vi "vipUninstall.vi"() -> ()   [LabVIEW 2014, in "lv-cli-steps.lvlib"]
uses:
  lv-cli-steps.lvlib
  <vilib>/Utility/error.llb/DialogType.ctl
  <vilib>/Wiresmith Technology/LabVIEW CLI/CLI Class/CLI.lvclass
  <vilib>/JKI/VIPM API/VIPM API_vipm_api.lvlib
panel:
  out "error out":errorcluster
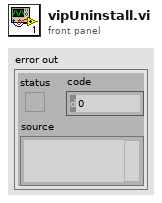
[diagram p1: front panel]
types:
  T1 = typedef "DialogType.ctl" = u16
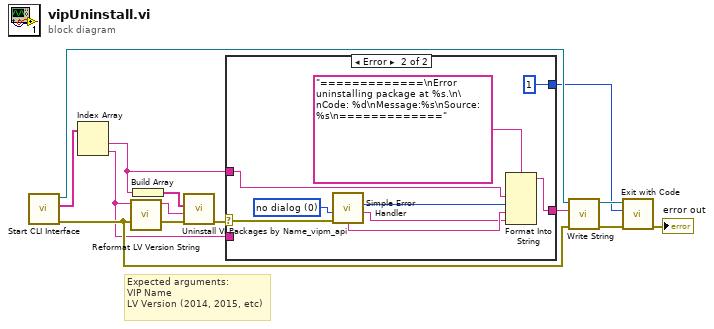
[diagram p0: block diagram]
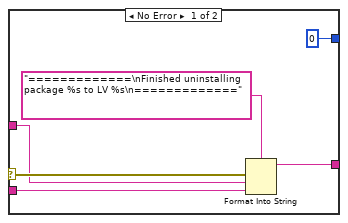
[diagram p2: hidden frame]
diagram:
  # "Expected arguments:\nVIP Name\nLV Version (2014, 2015, etc)"
  n1 = call <vilib>:"Start CLI Interface.vi"() -> ("error out"=w6:errorcluster, "Custom Parameters"=w13:string[], "CLI out"=w11:refnum<class "CLI.lvclass">)  [unwired: 9 in]
  n2 = Index Array(array=w13) -> (element #1=w4:string, element #2=w2:string)  [unwired: 2 in]
  n3 = call "Reformat LV Version String.vi"("Version String (2014)"=w2) -> ("Short Version String (14.0)"=w1:string)  [unwired: 10 in]
  n4 = Build Array(w4) -> (w3:string[])
  n5 = call <vilib>:"Uninstall VI Packages by Name_vipm_api.vi"("error in (no error)"=w6, "LabVIEW Version"=w1, "Package Names to Uninstall []"=w3) -> ("error out"=w5:errorcluster)  [unwired: 8 in]
  n6 = case shown="Error" w5 {
    selector: w5 -> [w18 w27]
    tunnel: w4 -> [w17 w23]
    tunnel: [w16 w28] -> w12
    tunnel: [0 ("Exit Code (0)") 1 ("Exit Code (0)")] -> w8
    tunnel: w2 -> [w14 _]
    frame No Error {
      n7 = Format Into String(format string="=============\nFinished uninstalling package %s to LV %s\n=============", error in=w18, w17, w14) -> (resulting string=w16:string)  [unwired: 1 in, 1 out]
    }
    frame Error {
      w26 = T1 0 items=["no dialog", "OK message", "continue or stop message", "OK message + warnings", "continue/stop + warnings"] ("type of dialog (OK msg:1)")
      n8 = call <vilib>:"Simple Error Handler.vi"("type of dialog (OK msg:1)"=w26, "error in (no error)"=w27) -> ("code out"=w20:i32, "source out"=w21:string, "message"=w22:string)  [unwired: 3 in, 2 out]
      n9 = Format Into String(format string="=============\nError uninstalling package at %s.\n\nCode: %d\nMessage:%s\nSource: %s\n=============", w23, w20, w22, w21) -> (resulting string=w28:string)  [unwired: 2 in, 1 out]
    }
  }
  n10 = call <vilib>:"Write String.vi"("error in (no error)"=w6, "Text to Write"=w12, "CLI in"=w11) -> ("error out"=w10:errorcluster, "CLI out"=w9:refnum<class "CLI.lvclass">)  [unwired: 7 in]
  n11 = call <vilib>:"Exit with Code.vi"("error in (no error)"=w10, "Exit Code (0)"=w8, "CLI in"=w9) -> ("error out"=→"error out":errorcluster)  [unwired: 8 in]
